vi "Configure Dialog.vi"(8 "error in (no error)":errorcluster, 11 "Configure Resume Trigger [RT] Msg in":refnum<class "Configure Resume Trigger [RT] Msg.lvclass">) -> (0 "error out":errorcluster, 2 "Ok?":bool, 3 "Configure Resume Trigger [RT] Msg out":refnum<class "Configure Resume Trigger [RT] Msg.lvclass">)   [LabVIEW 2014, in "CS++Fgen.lvlib" / "Configure Resume Trigger [RT] Msg.lvclass"]
uses:
  Configure Resume Trigger [RT] Msg.lvclass
  Configure Resume Trigger [RT] Msg.lvclass/Configure Resume Trigger [RT] Msg.ctl
panel:
  in  "Trigger Source (None)":string(combo) caption="Trigger Source"
  in  "Channel Name (\"\")":string="CHANNEL1" caption="Channel Name"
  in  "Trigger Slope (Positive)":i32(ring) caption="Trigger Slope" items=["Positive", "Negative", "Either"]
  in  "OK Button":bool
  in  "Cancel Button":bool
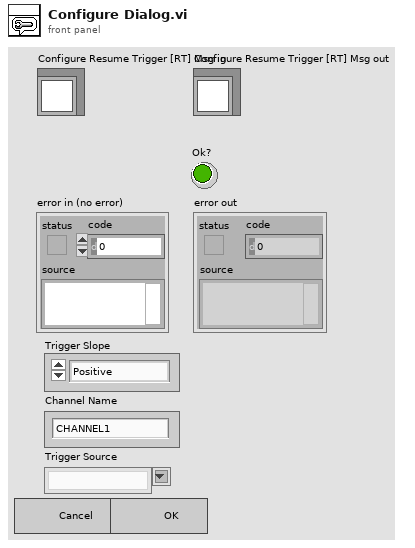
[diagram p1: front panel]
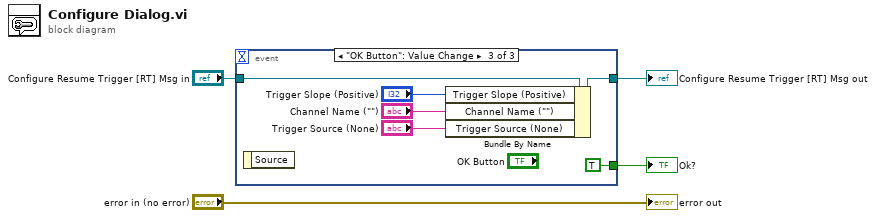
[diagram p0: block diagram]
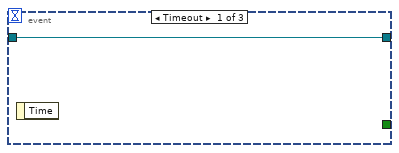
[diagram p2: hidden frame]
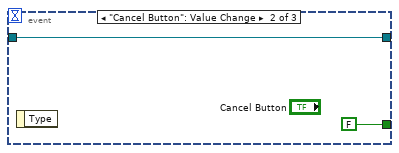
[diagram p3: hidden frame]
diagram:
  n1 = event shown="[2] \"OK Button\": Value Change" {
    selector: _ -> [_ _ _]
    dyn-events: _ -> [_ _ _]
    timeout: _ -> [_ _ _]
    tunnel: [w5 w7 w11] -> w3
    tunnel: "Configure Resume Trigger [RT] Msg in" -> [w5 w7 w13]
    tunnel: [_ FALSE TRUE] -> w1
    event Timeout {
      n2 = event-data() -> ()  [unwired: 1 in, 1 out]
    }
    event "Cancel Button": Value Change {
      n3 = event-data() -> ()  [unwired: 1 in, 1 out]
    }
    event "OK Button": Value Change {
      n4 = event-data() -> ()  [unwired: 1 in, 1 out]
      n5 = Bundle By Name(cluster=w13, "Trigger Slope (Positive)"="Trigger Slope (Positive)", "Channel Name (\"\")"="Channel Name (\"\")", "Trigger Source (None)"="Trigger Source (None)") -> (w11:refnum<class "Configure Resume Trigger [RT] Msg.lvclass">)
    }
  }
  "Configure Resume Trigger [RT] Msg out" <- w3
  "Ok?" <- w1
  "error out" <- "error in (no error)"
